vi "DRIVE_STRAIGHT_NAVX.vi"(10 "argv":string[](array[string]), 11 "args":u8) -> ()   [LabVIEW 2015]
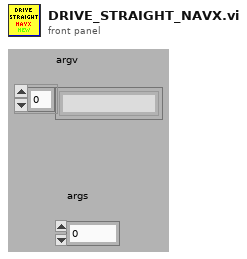
[diagram p1: front panel]
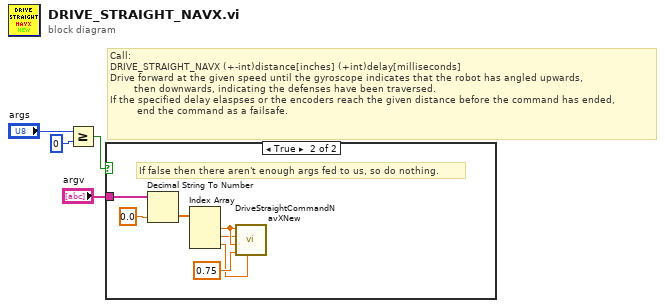
[diagram p0: block diagram]
diagram:
  # "Call:\nDRIVE_STRAIGHT_NAVX (+-int)distance[inches] (+int)delay[milliseconds]\nDrive forward at the given speed until the gyroscope indicates that the robot has angled upwards,\n        then downwards, indicating the defenses have been traversed.\nIf the specified delay elaspses or the encoders reach the given distance before the command has ended,\n         end the command as a failsafe."
  n1 = Greater Or Equal?(x="args", y=u8 0) -> (x >= y?=w4:bool)
  n2 = case shown="True" w4 {
    tunnel: "argv" -> [_ w11]
    frame False {
    }
    frame True {
      # "If false then there aren't enough args fed to us, so do nothing."
      n3 = Decimal String To Number(string=w11, default (0L)=0.0 ("default (0 I32)")) -> (number=w8:dbl[])  [unwired: 2 out]
      n4 = Index Array(array=w8) -> (element #1=w7:dbl, element #2=w6:dbl, element #3=w5:dbl)  [unwired: 3 in]
      n5 = call "DriveStraightCommandNavXNew.vi"("Flat Delay"=w5, "speed"=0.75, "Fwd Bwd"=w7, "Delay ms"=w6, "distance"=w7) -> ()  [unwired: 7 in]
    }
  }
